vi "galvo.scan.engine_MD.vi"   [LabVIEW 2012]
uses:
  <vilib>/Utility/VariantDataType/Type.ctl
  Custom Controls/scan mode main settings tab.ctl
  <vilib>/DAQmx/write.llb/DAQmx Write (Analog 1D Wfm NChan NSamp).vi
  <vilib>/DAQmx/read.llb/DAQmx Read (Analog 2D I16 NChan NSamp).vi
  GFG/GFGnumericGet.vi
  GFG/GFGstringGet.vi
  GFG/GFGbooleanGet.vi
  <vilib>/Waveform/WDTOps.llb/WDT Number of Waveform Samples DBL.vi
  <vilib>/DAQmx/configure/timing.llb/DAQmx Timing (Sample Clock).vi
  <vilib>/DAQmx/configure/trigger.llb/DAQmx Start Trigger (Digital Edge).vi
  <vilib>/DAQmx/create/channels.llb/DAQmx Create Channel (AO-Voltage-Basic).vi
  <vilib>/DAQmx/configure/timing.llb/DAQmx Timing (Use Waveform).vi
  <vilib>/DAQmx/miscellaneous.llb/DAQmx Fill In Error Info.vi
  GFG/GFGfpRefGet.vi
  <resource>/objmgr/daqmx.rc
  GFG/GFG library.lvlib
  <vilib>/Utility/VariantDataType/VariantType.lvlib
types:
  T1 = typedef "scan mode main settings tab.ctl" = enum32{"2D frame", "2D line scan", "general settings", "Z Stack", "piezo"}
  T2 = enum8{"Enabled", "Disabled", "Disabled and Grayed Out"}
  T3 = cluster{"WaveformChartRef":refnum<vi>, "DigitalRef":refnum<vi>, "ArrayRef":refnum<vi>, "TabControlRef":refnum<vi>, "EnumRef":refnum<vi>, "RingRef":refnum<vi>, "BooleanRef":refnum<vi>, "KnobRef":refnum<vi>, "SlideRef":refnum<vi>, "PathRef":refnum<vi>, "StringRef":refnum<vi>, "ComboBox":refnum<vi>, "WaveformGraphRef":refnum<vi>}
  T4 = cluster{"NewVal":bool, "Event Registration Refnum":refnum<event-registration>}
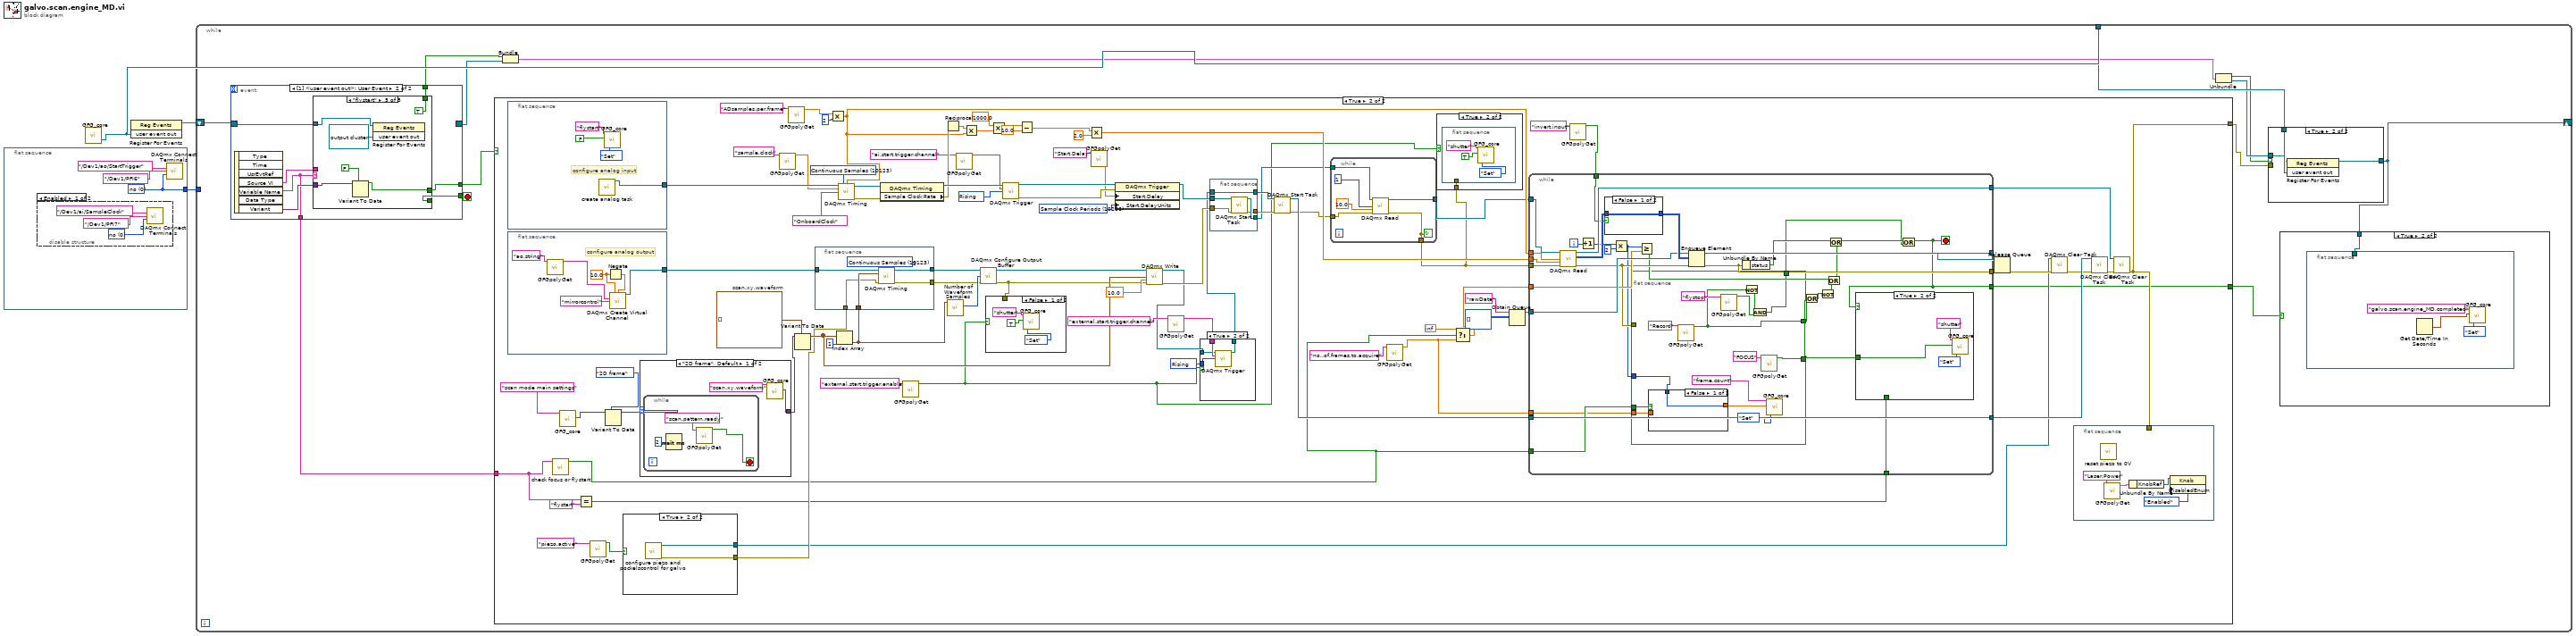
[diagram p0: block diagram]
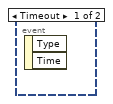
[diagram p5: hidden frame]
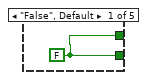
[diagram p6: hidden frame]
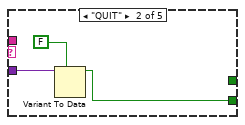
[diagram p7: hidden frame]
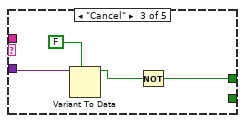
[diagram p8: hidden frame]
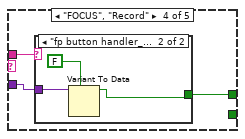
[diagram p9: hidden frame]
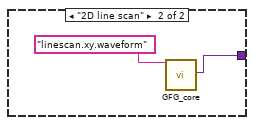
[diagram p16: hidden frame]
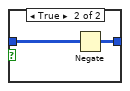
[diagram p17: hidden frame]
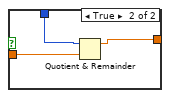
[diagram p18: hidden frame]
diagram:
  n1 = flat-sequence {
    tunnel: [w4] -> w3
    frame #0 {
      w4 = 0 items=["no", "yes"] ("invert polarity")
      n2 = disable-structure shown="Enabled" {
        frame Enabled {
          w9 = 0 items=["no", "yes"] ("invert polarity")
          n3 = call <vilib>:"DAQmx Connect Terminals.vi"("source terminal"=tag "/Dev1/ai/SampleClock", "destination terminal"=tag "/Dev1/PFI7", "invert polarity"=w9) -> ()  [unwired: 12 in, 1 out]
        }
        frame Disabled {
        }
      }
      n4 = call <vilib>:"DAQmx Connect Terminals.vi"("source terminal"=tag "/Dev1/ao/StartTrigger", "destination terminal"=tag "/Dev1/PFI6", "invert polarity"=w4) -> ()  [unwired: 12 in, 1 out]
    }
  }
  n5 = call "GFG_core.vi"() -> ("user event out"=w1:refnum<user-event>)  [unwired: 13 in, 6 out]
  n6 = register-events(w1) -> (reference out=w2:refnum<event-registration>)  [unwired: 2 in, 1 out]
  n7 = while {
    tunnel: w3 -> [_]
    tunnel: w1 -> [w19]
    shift-right: [w16] -> _
    shift-left: w2 -> [w20]
    stop <- w21 stop-if-true
    n8 = event shown="[1] <user event out>: User Event" {
      selector: w20 -> [_ w33]
      dyn-events: [_ _] -> w15
      timeout: _ -> [_ _]
      tunnel: [_ w37] -> w22
      tunnel: [_ w36] -> w21
      tunnel: [_ w32] -> w18
      tunnel: [_ w31] -> w14
      event Timeout {
        n9 = event-data() -> ()  [unwired: 1 in, 2 out]
      }
      event User Event {
        n10 = event-data() -> ("Source VI"=w34:string, "Variable Name"=w32:string, "Variant"=w35:variant)  [unwired: 1 in, 4 out]
        n11 = case shown="\"flystart\"" w32 {
          tunnel: [w38 _ w42 w47 w55] -> w37
          tunnel: [w38 w39 _ _ _] -> w36
          tunnel: w35 -> [_ w41 w44 w48 w56]
          tunnel: w34 -> [_ _ _ w46 _]
          tunnel: w33 -> [_ _ _ _ w53]
          tunnel: [_ _ _ _ TRUE ("NewVal")] -> w31
          frame "False", Default {
            w38 = FALSE ("NewVal")
          }
          frame "QUIT" {
            n12 = Variant To Data(type=FALSE ("NewVal"), Variant=w41) -> (data=w39:bool)  [unwired: 1 in, 1 out]
          }
          frame "Cancel" {
            n13 = Variant To Data(type=FALSE ("NewVal"), Variant=w44) -> (data=w43:bool)  [unwired: 1 in, 1 out]
            n14 = Not(x=w43) -> (.not. x?=w42:bool)
          }
          frame "FOCUS", "Record" {
            n15 = case shown="\"fp button handler_MD.vi\"" w46 {
              tunnel: w48 -> [_ w50]
              tunnel: [_ w49] -> w47
              frame "False", Default {
              }
              frame "fp button handler_MD.vi" {
                n16 = Variant To Data(type=FALSE ("NewVal"), Variant=w50) -> (data=w49:bool)  [unwired: 1 in, 1 out]
              }
            }
          }
          frame "flystart" {
            n17 = Variant To Data(type=FALSE ("NewVal"), Variant=w56) -> (data=w55:bool)  [unwired: 1 in, 1 out]
            n18 = register-events(reference=w53, refnum<user-event> refnum ("user event out")) -> ()  [unwired: 1 in, 2 out]
          }
        }
      }
    }
    n19 = case shown="True" w22 {
      tunnel: [_ w68] -> w17
      tunnel: w18 -> [_ w59]
      tunnel: [_ w60] -> w10
      frame False {
      }
      frame True {
        w85 = 10280 items=["Rising"=10280, "Falling"=10171] ("Slope")
        w105 = waveform(dbl)[] []  # scan.xy.waveform
        w139 = 10280 items=["Rising"=10280, "Falling"=10171] ("Slope")
        w116 = 10286 items=["Sample Clock Periods"=10286, "Seconds"=10364, "Ticks"=10304] ("Start.DelayUnits")
        w143 = 10123 items=["Finite Samples"=10178, "Continuous Samples"=10123] ("sample mode")
        n20 = flat-sequence {
          tunnel: [w196] -> w142
          frame #0 {
            # "configure analog input"
            n21 = call "create analog task.vi"() -> ("task out"=w196:refnum<k21>)  [unwired: 11 in]
            n22 = call "GFG_core.vi"("Variable Name in"="flystart", "Variant in"=FALSE ("NewVal"), "Action"=enum16{"Init", "Set", "Get"}."Set") -> ()  [unwired: 10 in, 7 out]
          }
        }
        n23 = flat-sequence {
          tunnel: [w191] -> w141
          frame #0 {
            w189 = 10.0 ("maximum value")
            # "configure analog output"
            n24 = call-poly "GFGpolyGet.vi"("Variable Name in"="ao.string" ("name to assign")) -> ("String"=w187:string)  [unwired: 10 in]
            n25 = Negate(x=w189) -> (-x=w190:dbl)
            n26 = call-poly <vilib>:"DAQmx Create Virtual Channel.vi"("maximum value"=w189, "minimum value"=w190, "physical channels"=w187, "name to assign"="mirrorcontrol") -> ("task out"=w191:refnum<k21>)  [unwired: 10 in, 1 out]
          }
        }
        n27 = call "check focus or flystart.vi"("x"=w59) -> ("x .or. y?"=w58:bool)  [unwired: 10 in]
        n28 = call "GFG_core.vi"("Variable Name in"="scan mode main settings") -> ("Variant Out"=w89:variant)  [unwired: 12 in, 6 out]
        n29 = Equal?(x=w59, y="flystart") -> (x = y?=w61:bool)
        n30 = call-poly "GFGpolyGet.vi"("Variable Name in"="piezo.active") -> ("Boolean"=w73:bool)  [unwired: 10 in]
        n31 = Variant To Data(type=scan_mode_main_settings_tab."2D frame" ("scan mode main settings"), Variant=w89) -> (data=w87:T1)  [unwired: 1 in, 1 out]
        n32 = case shown="True" w73 {
          tunnel: [_ w154] -> w72
          tunnel: [_ w153] -> w69
          frame False {
          }
          frame True {
            n33 = call "configure piezo and pockelscontrol for galvo.vi"() -> ("error out"=w154:errorcluster, "task out"=w153:refnum<k21>)  [unwired: 10 in]
          }
        }
        n34 = case shown="\"2D frame\", Default" w87 {
          tunnel: [w175 w180] -> w104
          frame "2D frame", Default {
            n35 = while {
              stop <- w178 stop-if-true
              n36 = Wait (ms)(milliseconds to wait=u32 2) -> ()  [unwired: 1 out]
              n37 = call-poly "GFGpolyGet.vi"("Variable Name in"="scan.pattern.ready") -> ("Boolean"=w178:bool)  [unwired: 10 in]
            }
            n38 = call "GFG_core.vi"("Variable Name in"="scan.xy.waveform") -> ("Variant Out"=w175:variant)  [unwired: 12 in, 6 out]
          }
          frame "2D line scan" {
            n39 = call "GFG_core.vi"("Variable Name in"="linescan.xy.waveform") -> ("Variant Out"=w180:variant)  [unwired: 12 in, 6 out]
          }
        }
        n40 = call-poly "GFGpolyGet.vi"("Variable Name in"="sample.clock" ("Tag in")) -> ("Numeric"=w120:dbl)  [unwired: 9 in, 1 out]
        n41 = call-poly "GFGpolyGet.vi"("Variable Name in"="ADsamples.per.frame" ("Tag in")) -> ("Numeric"=w122:dbl)  [unwired: 9 in, 1 out]
        n42 = Variant To Data(type=w105, Variant=w104) -> (data=w103:waveform(dbl)[])  [unwired: 1 in, 1 out]
        n43 = flat-sequence {
          tunnel: w141 -> [w159]
          tunnel: w125 -> [w158]
          tunnel: [w157] -> w118
          tunnel: [w156] -> w94
          tunnel: w72 -> [w155]
          frame #0 {
            w160 = 10123 items=["Finite Samples"=10178, "Continuous Samples"=10123] ("sample mode")
            n44 = call-poly <vilib>:"DAQmx Timing.vi"("task/channels in"=w159, "sample mode"=w160, "waveform"=w158, "error in"=w155) -> ("task out"=w157:refnum<k21>, "error out"=w156:errorcluster)  [unwired: 10 in]
          }
        }
        n45 = Multiply(x=w122, y=i8 2) -> (x*y=w110:dbl)
        n46 = Index Array(array=w103, index=1) -> (element=w125:waveform(dbl))
        n47 = call-poly <vilib>:"DAQmx Timing.vi"("task/channels in"=w142, "sample mode"=w143, "samples per channel"=w110, "rate"=w120, "source"=tag "OnboardClock") -> ("task out"=w115:refnum<k21>, "error out"=w114:errorcluster)  [unwired: 9 in]
        n48 = property class="DAQmx Timing"(reference=w115, error in=w114) -> (reference out=w113:refnum<k21>, "Sample Clock:Rate"=w112:dbl)  [unwired: 1 out]
        n49 = call-poly "GFGpolyGet.vi"("Variable Name in"="external.start.trigger.enable" ("Tag in")) -> ("Boolean"=w63:bool)  [unwired: 10 in]
        n50 = Reciprocal(x=w112) -> (1/x=w111:dbl)
        n51 = call-poly <vilib>:"Number of Waveform Samples.vi"("waveform in"=w125) -> ("number of samples"=w128:i32)  [unwired: 8 in, 2 out]
        n52 = call-poly "GFGpolyGet.vi"("Variable Name in"="ai.start.trigger.channel" ("Tag in")) -> ("String"=w106:string)  [unwired: 10 in]
        n53 = Multiply(x=w111, y=w110) -> (x*y=w109:dbl)
        n54 = call <vilib>:"DAQmx Configure Output Buffer.vi"("task/channels in"=w118, "buffer size (in samples per channel)"=w128, "error in"=w94) -> ("task out"=w133:refnum<k21>, "error out"=w75:errorcluster)  [unwired: 11 in]
        n55 = case shown="False" w63 {
          tunnel: w75 -> [_ _]
          frame False {
            n56 = call "GFG_core.vi"("Variable Name in"="shutter" ("Tag in"), "Variant in"=TRUE, "Action"=enum16{"Init", "Set", "Get"}."Set") -> ()  [unwired: 10 in, 7 out]
          }
          frame True {
          }
        }
        n57 = Multiply(x=1000.0, y=w109) -> (x*y=w98:dbl)
        n58 = call-poly <vilib>:"DAQmx Trigger.vi"("task/channels in"=w113, "source"=w106, "edge"=w139) -> ("task out"=w138:refnum<k21>, "error out"=w137:errorcluster)  [unwired: 11 in]
        n59 = Subtract(x=w98, y=10.0) -> (x-y=w99:dbl)
        n60 = Multiply(x=w99, y=2.0) -> (x*y=w96:dbl)
        n61 = call-poly "GFGpolyGet.vi"("Variable Name in"="Start.Delay" ("Tag in")) -> ("Numeric"=w117:dbl)  [unwired: 9 in, 1 out]
        n62 = property class="DAQmx Trigger"(reference=w138, error in=w137, "Start.Delay"=w117, "Start.DelayUnits"=w116) -> (reference out=w126:refnum<k21>)  [unwired: 1 out]
        n63 = call-poly <vilib>:"DAQmx Write.vi"("task/channels in"=w133, "data"=w103, "timeout"=10.0 ("Wirite Timeout"), "error in"=w75) -> ("task out"=w83:refnum<k21>, "error out"=w93:errorcluster)  [unwired: 9 in, 1 out]
        n64 = call-poly "GFGpolyGet.vi"("Variable Name in"="external.start.trigger.channel" ("Tag in")) -> ("String"=w86:string)  [unwired: 10 in]
        n65 = case shown="True" w63 {
          tunnel: w86 -> [_ w174]
          tunnel: w85 -> [_ w173]
          tunnel: w83 -> [w170 w172]
          tunnel: [w170 w171] -> w82
          frame False {
          }
          frame True {
            n66 = call-poly <vilib>:"DAQmx Trigger.vi"("task/channels in"=w172, "source"=w174, "edge"=w173) -> ("task out"=w171:refnum<k21>)  [unwired: 11 in, 1 out]
          }
        }
        n67 = flat-sequence {
          tunnel: w126 -> [w186]
          tunnel: [w185] -> w78
          tunnel: [w184] -> w102
          tunnel: w82 -> [w183]
          tunnel: [w183] -> w101
          tunnel: w93 -> [w182]
          frame #0 {
            n68 = call <vilib>:"DAQmx Start Task.vi"("task/channels in"=w186, "error in"=w182) -> ("task out"=w185:refnum<k21>, "error out"=w184:errorcluster)  [unwired: 12 in]
          }
        }
        n69 = call <vilib>:"DAQmx Start Task.vi"("task/channels in"=w101, "error in"=w102) -> ("task out"=w80:refnum<k21>, "error out"=w79:errorcluster)  [unwired: 12 in]
        n70 = while {
          tunnel: w79 -> [w164]
          tunnel: w78 -> [w163]
          tunnel: [w162] -> w77
          tunnel: [w161] -> w76
          stop <- w161 continue-if-true
          n71 = call-poly <vilib>:"DAQmx Read.vi"("task/channels in"=w163, "number of samples per channel"=1, "timeout"=10.0, "error in"=w164) -> ("task out"=w162:refnum<k21>, "error out"=w161:errorcluster)  [unwired: 9 in, 1 out]
        }
        n72 = call-poly "GFGpolyGet.vi"("Variable Name in"="no..of.frames.to.acquire" ("Tag in")) -> ("Numeric"=w64:dbl)  [unwired: 9 in, 1 out]
        n73 = case shown="True" w63 {
          tunnel: w76 -> [_ w145]
          frame False {
          }
          frame True {
            n74 = flat-sequence {
              tunnel: w145 -> [_]
              frame #0 {
                n75 = call "GFG_core.vi"("Variable Name in"="shutter" ("Tag in"), "Variant in"=TRUE, "Action"=enum16{"Init", "Set", "Get"}."Set") -> ()  [unwired: 10 in, 7 out]
              }
            }
          }
        }
        n76 = Select(t=inf, s=w58, f=w64) -> (s? t:f=w65:dbl)
        n77 = Obtain Queue(name (unnamed)="rawData", element data type=i16[][] [] ("-x")) -> (queue out=w130:refnum<queue>)  [unwired: 3 in, 2 out]
        n78 = call-poly "GFGpolyGet.vi"("Variable Name in"="invert.input" ("Tag in")) -> ("Boolean"=w91:bool)  [unwired: 10 in]
        n79 = while {
          tunnel: [w220] -> w144
          tunnel: w80 -> [w227]
          tunnel: [w227] -> w140
          tunnel: [w219] -> w100
          tunnel: w110 -> [w222]
          tunnel: w130 -> [w225]
          tunnel: [w224] -> w129
          tunnel: w65 -> [w221]
          tunnel: w96 -> [w214]
          tunnel: w76 -> [w210]
          tunnel: w91 -> [w209]
          tunnel: w77 -> [w207]
          tunnel: w58 -> [w203]
          tunnel: w64 -> [w202]
          tunnel: w61 -> [w201]
          tunnel: [w197] -> w60
          i -> [w218]
          stop <- w197 stop-if-true
          n80 = call-poly <vilib>:"DAQmx Read.vi"("task/channels in"=w207, "number of samples per channel"=w222, "timeout"=w214, "error in"=w210) -> ("task out"=w220:refnum<k21>, "data"=w223:i16[][], "error out"=w211:errorcluster)  [unwired: 9 in]
          n81 = Increment(x=w218) -> (x+1=w213:i32)
          n82 = case shown="False" w209 {
            tunnel: [w228 w230] -> w226
            tunnel: w223 -> [w228 w229]
            frame False {
            }
            frame True {
              n83 = Negate(x=w229) -> (-x=w230:i16[][])
            }
          }
          n84 = Multiply(x=w213, y=2) -> (x*y=w208:i32)
          n85 = flat-sequence {
            tunnel: [w242] -> w199
            tunnel: [w232] -> w217
            tunnel: w211 -> [_]
            tunnel: w208 -> [w237]
            tunnel: w203 -> [w240]
            tunnel: w202 -> [w238]
            tunnel: [w231] -> w198
            frame #0 {
              n86 = case shown="False" w240 {
                tunnel: w238 -> [_ w248]
                tunnel: w237 -> [w245 w247]
                tunnel: [w245 w246] -> w236
                frame False {
                }
                frame True {
                  n87 = Quotient & Remainder(x=w247, y=w248) -> (x-y*floor(x/y)=w246:dbl)  [unwired: 1 out]
                }
              }
              n88 = call-poly "GFGpolyGet.vi"("Variable Name in"="Record") -> ("Boolean"=w232:bool)  [unwired: 10 in]
              n89 = call-poly "GFGpolyGet.vi"("Variable Name in"="flystop") -> ("Boolean"=w233:bool)  [unwired: 10 in]
              n90 = Not(x=w232) -> (.not. x?=w234:bool)
              n91 = And(x=w234, y=w233) -> (x .and. y?=w231:bool)
              n92 = call-poly "GFGpolyGet.vi"("Variable Name in"="FOCUS") -> ("Boolean"=w242:bool)  [unwired: 10 in]
              n93 = call "GFG_core.vi"("Variable Name in"="frame.count", "Variant in"=w236, "Action"=enum16{"Init", "Set", "Get"}."Set") -> ()  [unwired: 10 in, 7 out]
            }
          }
          n94 = Greater Or Equal?(x=w208, y=w221) -> (x >= y?=w205:bool)
          n95 = Enqueue Element(queue=w225, element=w226, error in (no error)=w211) -> (queue out=w224:refnum<queue>, error out=w219:errorcluster)  [unwired: 1 in, 1 out]
          n96 = Unbundle By Name(w219) -> ("status"=w206:bool)
          n97 = Or(x=w217, y=w199) -> (x .or. y?=w216:bool)
          n98 = Not(x=w216) -> (.not. x?=w215:bool)
          n99 = Or(x=w205, y=w215) -> (x .or. y?=w204:bool)
          n100 = Or(x=w206, y=w204) -> (x .or. y?=w200:bool)
          n101 = Or(x=w200, y=w198) -> (x .or. y?=w197:bool)
          n102 = case shown="True" w197 {
            tunnel: w201 -> [_ _]
            tunnel: w199 -> [_ w249]
            frame False {
            }
            frame True {
              n103 = call "GFG_core.vi"("Variable Name in"="shutter" ("Tag in"), "Variant in"=w249, "Action"=enum16{"Init", "Set", "Get"}."Set") -> ()  [unwired: 10 in, 7 out]
            }
          }
        }
        n104 = Release Queue(queue=w129, error in (no error)=w100) -> (error out=w71:errorcluster)  [unwired: 1 in, 2 out]
        n105 = call <vilib>:"DAQmx Clear Task.vi"("task in"=w69, "error in"=w71) -> ("error out"=w70:errorcluster)  [unwired: 13 in]
        n106 = flat-sequence {
          tunnel: w68 -> [_]
          frame #0 {
            n107 = call "reset piezo to 0V.vi"() -> ()  [unwired: 11 in, 1 out]
            n108 = call-poly "GFGpolyGet.vi"("Variable Name in"="Laser.Power") -> ("output cluster"=w152:T3)  [unwired: 9 in, 1 out]
            n109 = Unbundle By Name(w152) -> ("KnobRef"=w149:refnum<vi>)
            n110 = property class="Knob"(reference=w149, "DisabledEnum"=T2."Enabled" ("Disabled")) -> ()  [unwired: 1 in, 2 out]
          }
        }
        n111 = call <vilib>:"DAQmx Clear Task.vi"("task in"=w140, "error in"=w70) -> ("error out"=w134:errorcluster)  [unwired: 13 in]
        n112 = call <vilib>:"DAQmx Clear Task.vi"("task in"=w144, "error in"=w134) -> ("error out"=w68:errorcluster)  [unwired: 13 in]
      }
    }
    n113 = Bundle("NewVal"=w14, "Event Registration Refnum"=w15) -> (w13:T4)  [unwired: 1 in]
    n114 = Unbundle(w13) -> ("NewVal"=w11:bool, "Event Registration Refnum"=w12:refnum<event-registration>)
    n115 = case shown="True" w11 {
      tunnel: w19 -> [_ w26]
      tunnel: w17 -> [_ _]
      tunnel: [w23 w25] -> w16
      tunnel: w12 -> [w23 w24]
      frame False {
      }
      frame True {
        n116 = register-events(reference=w24, w26) -> (reference out=w25:refnum<event-registration>)  [unwired: 1 in, 1 out]
      }
    }
    n117 = case shown="True" w10 {
      tunnel: w16 -> [_ w27]
      frame False {
      }
      frame True {
        n118 = flat-sequence {
          tunnel: w27 -> [_]
          frame #0 {
            n119 = Get Date/Time In Seconds() -> (seconds since 1Jan1904=w28:timestamp)
            n120 = call "GFG_core.vi"("Variable Name in"="galvo.scan.engine_MD.completed", "Variant in"=w28, "Action"=enum16{"Init", "Set", "Get"}."Set") -> ()  [unwired: 10 in, 7 out]
          }
        }
      }
    }
  }
